vi "Sistema_Aquisicao.vi"() -> ()   [LabVIEW 2012]
uses:
  Global_Telescopio.vi
panel:
  out "error out":errorcluster
  out "ultimo valor 2":dbl format="%#_9g"
  out "ultimo valor":dbl format="%#_9g"
  out "ultimo comando":dbl
  in  "Case Constant\n(See Context Help)":bool=TRUE
  out "O Recebido":bool
  out "TimeoutAq":u32
  out "concatenated string":string
  out "Maq Satus":i32
  out "TX":string
  out "Serial Settings:Number of Bytes at Serial Port":u32
  out "Data rx Aquisição":string
  # "2"
  # "R -->Registra Centragem\nS -->Status\nO -->OffSet\nF ---> Foco"
  # "3"
  # "4"
  # "5"
  # "!"
  # "!"
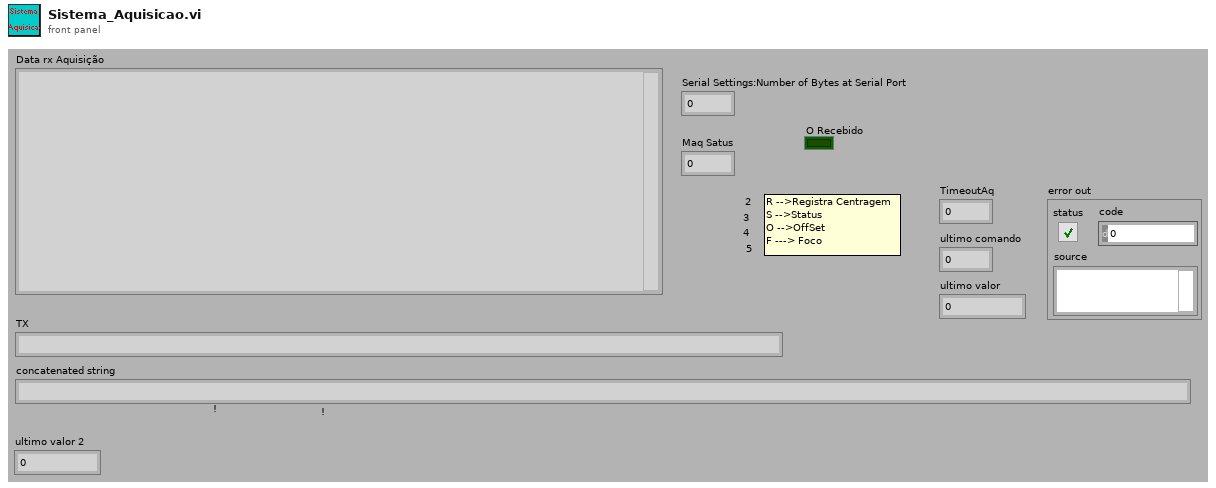
[diagram p1: front panel]
types:
  T1 = enum16{"open", "open or create", "create or replace", "create"}
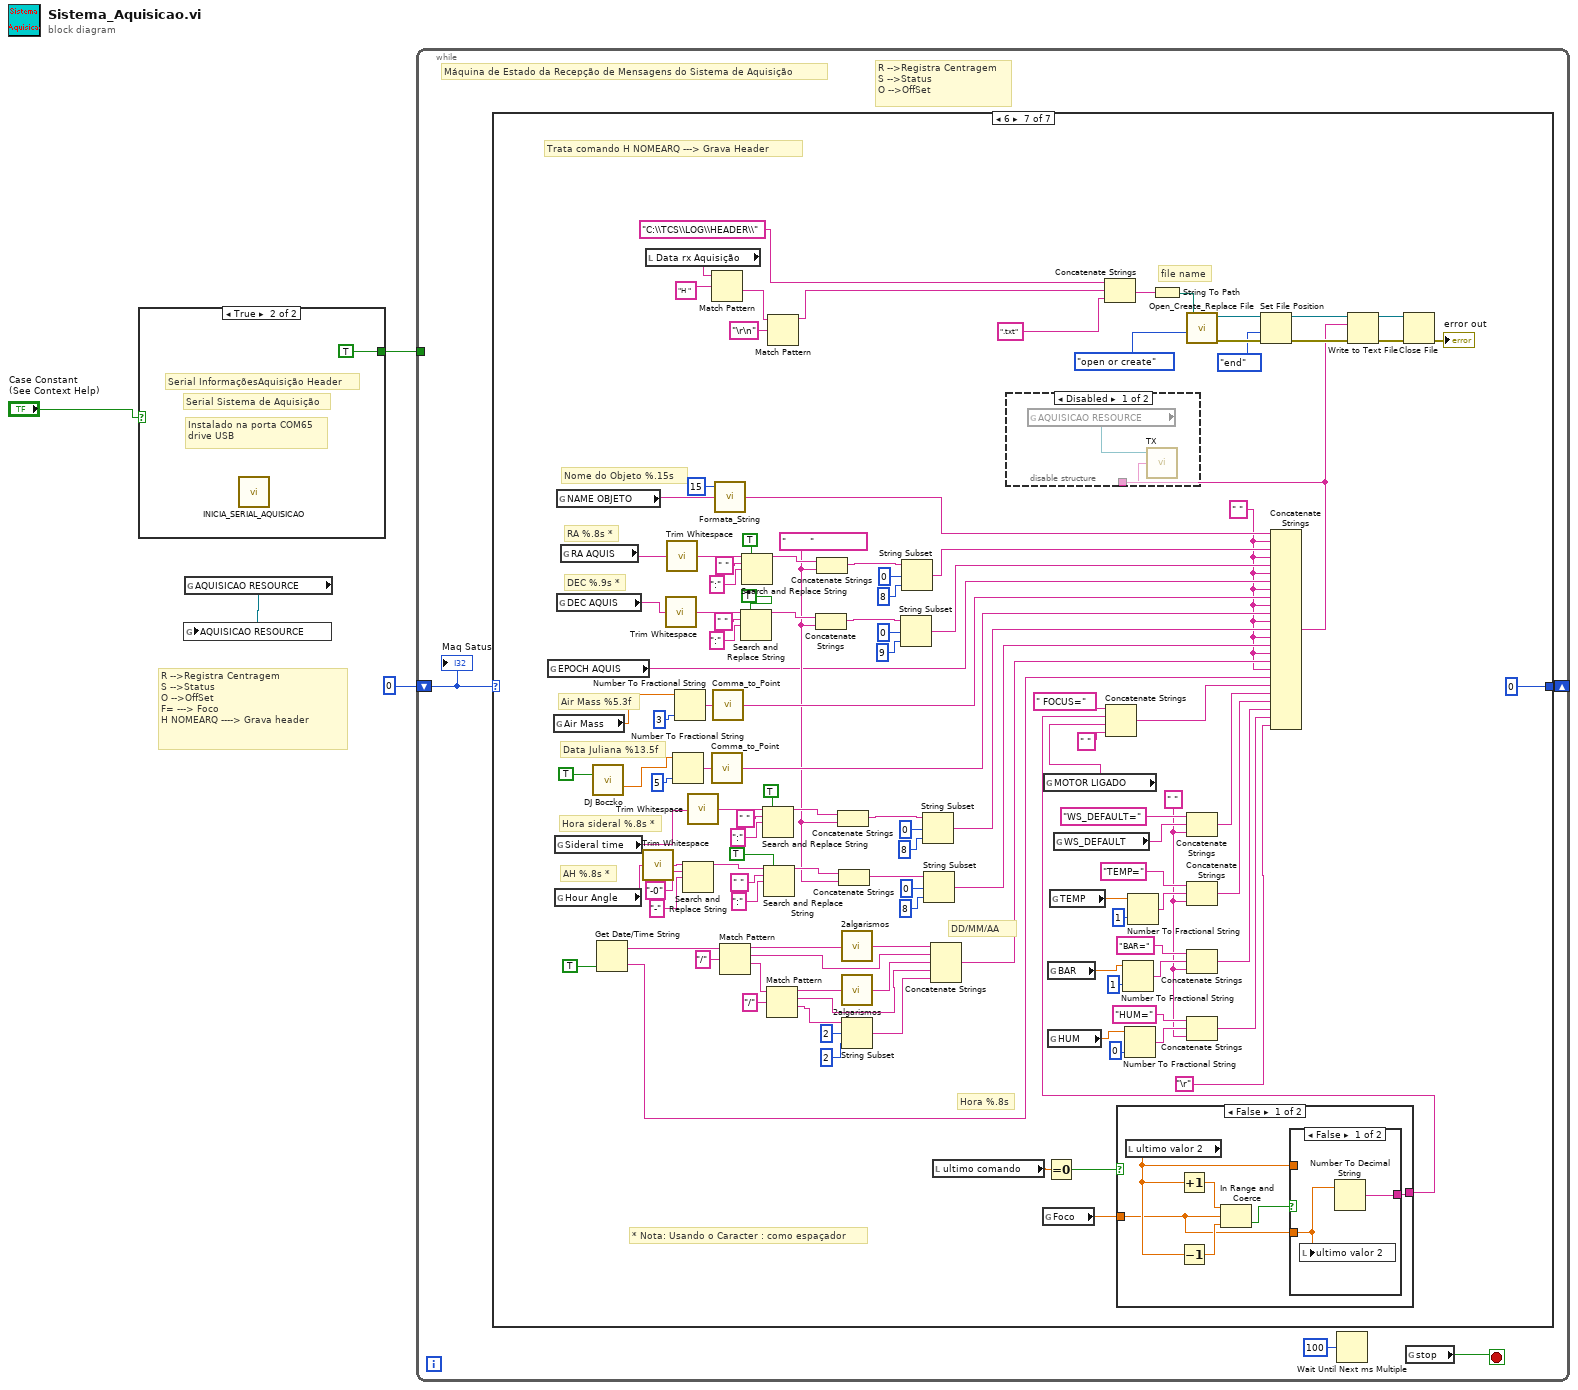
[diagram p0: block diagram]
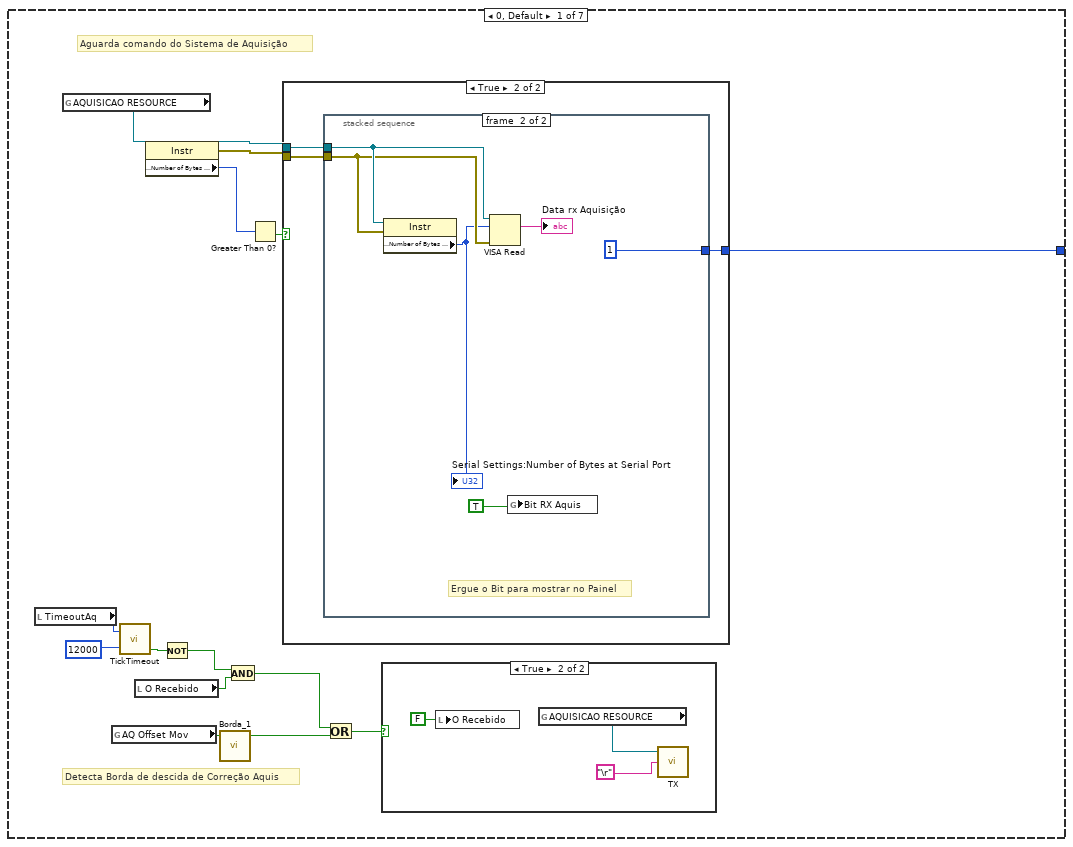
[diagram p3: hidden frame]
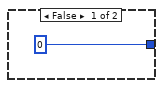
[diagram p5: hidden frame]
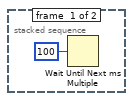
[diagram p6: hidden frame]
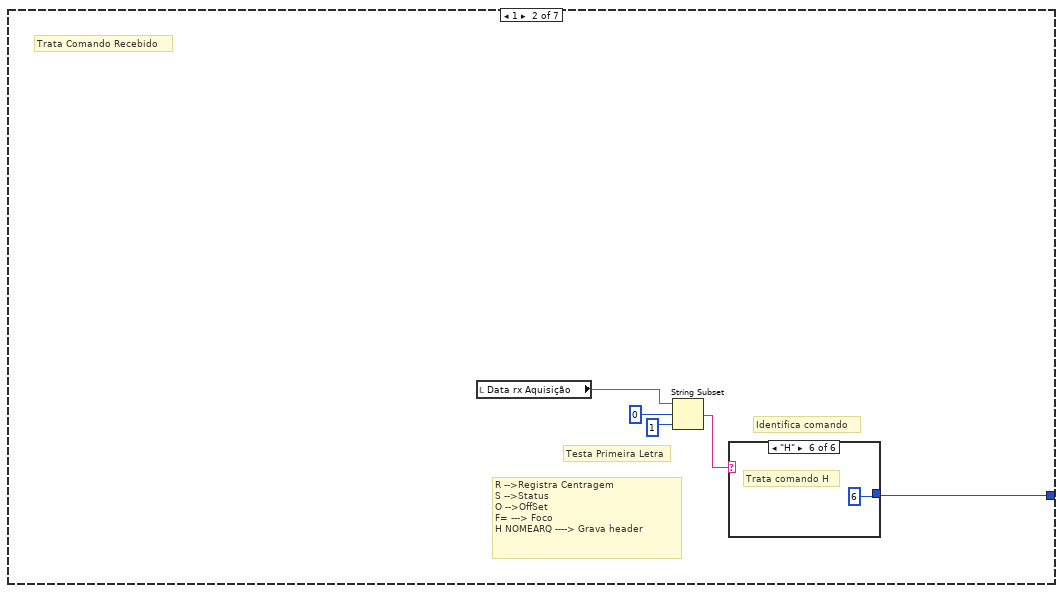
[diagram p7: hidden frame]
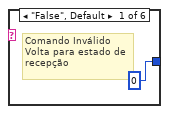
[diagram p8: hidden frame]
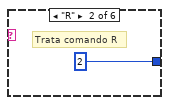
[diagram p9: hidden frame]
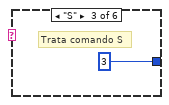
[diagram p10: hidden frame]
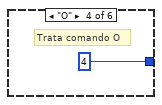
[diagram p11: hidden frame]
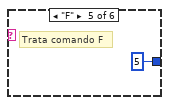
[diagram p12: hidden frame]
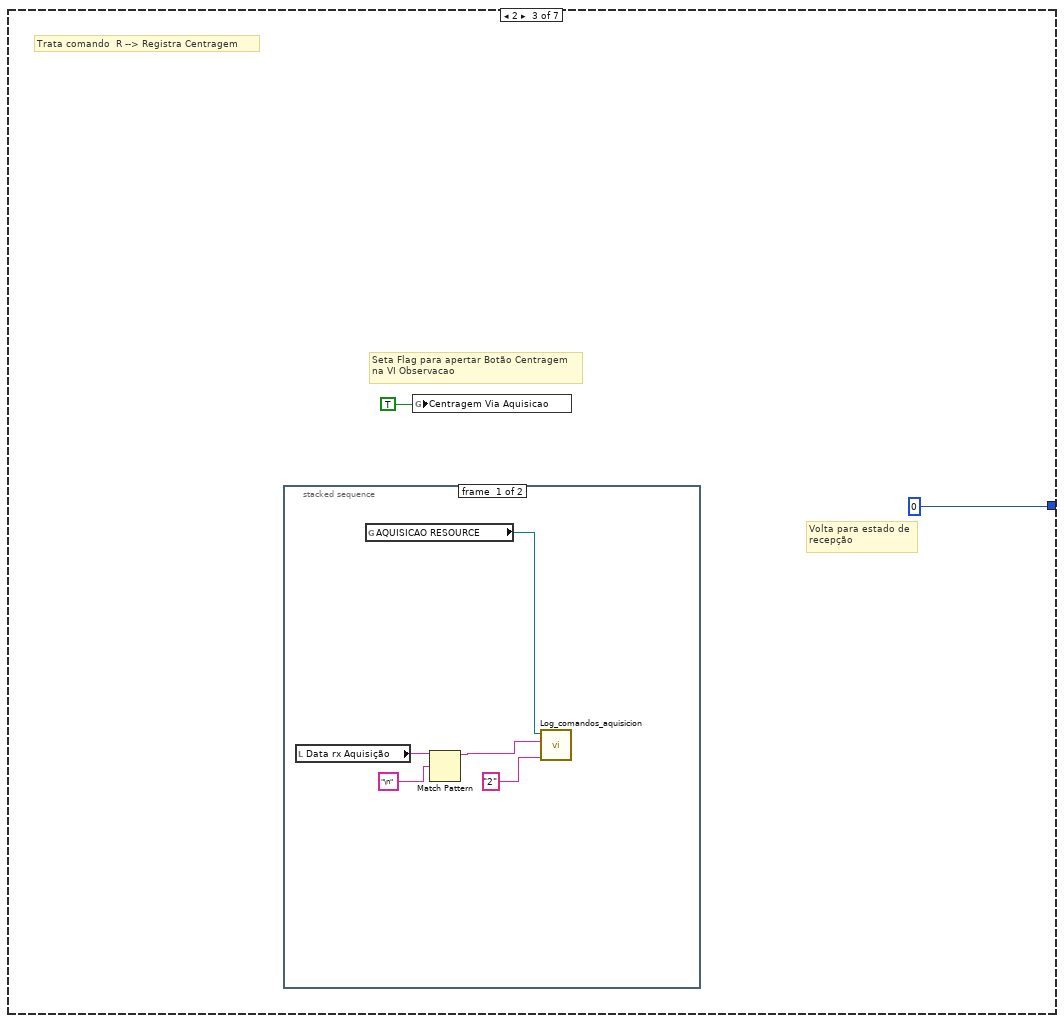
[diagram p13: hidden frame]
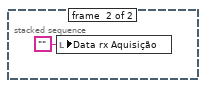
[diagram p14: hidden frame]
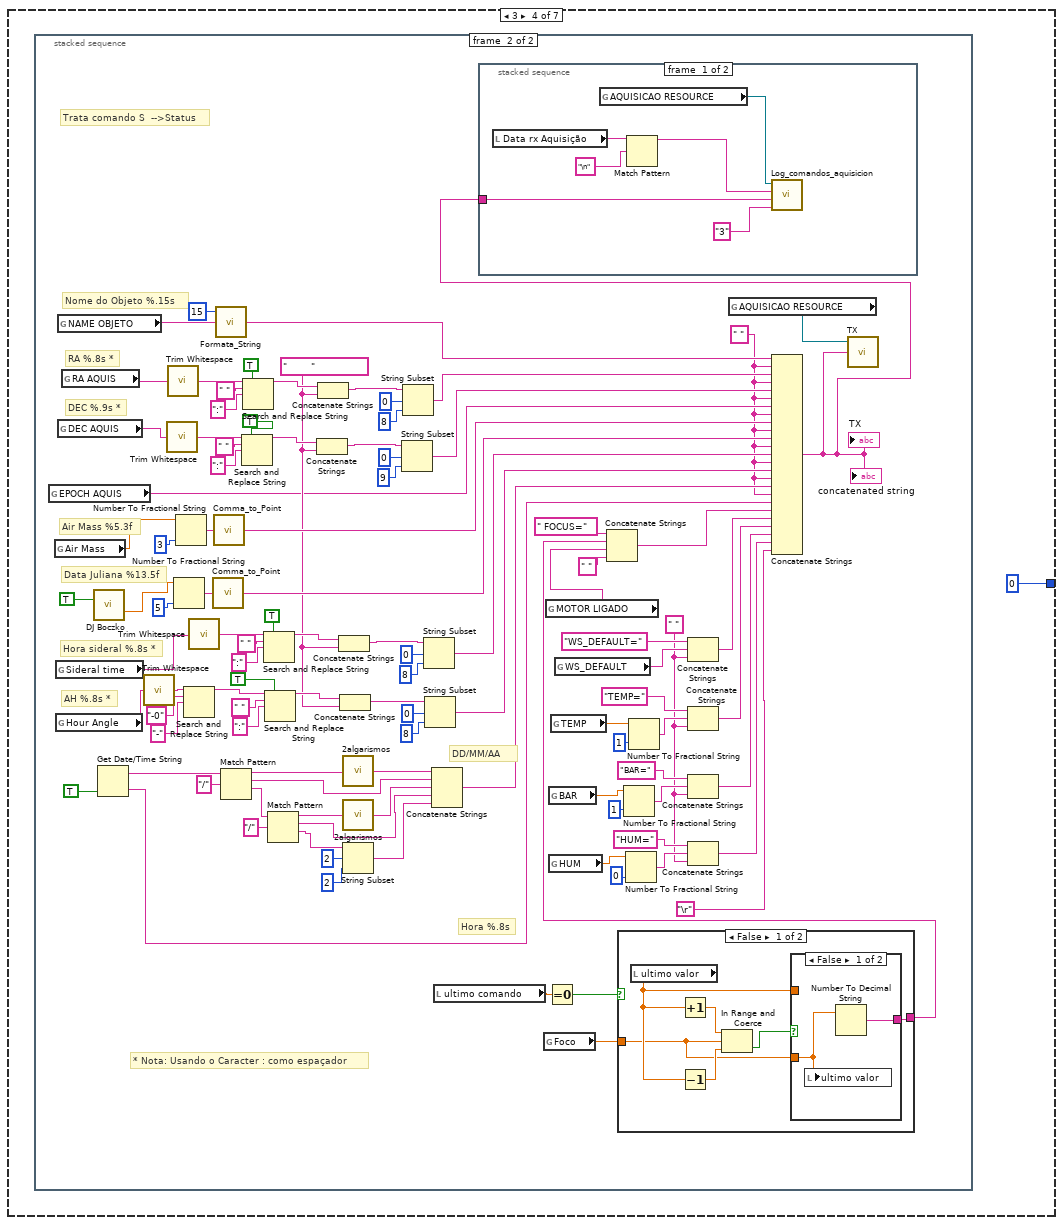
[diagram p15: hidden frame]
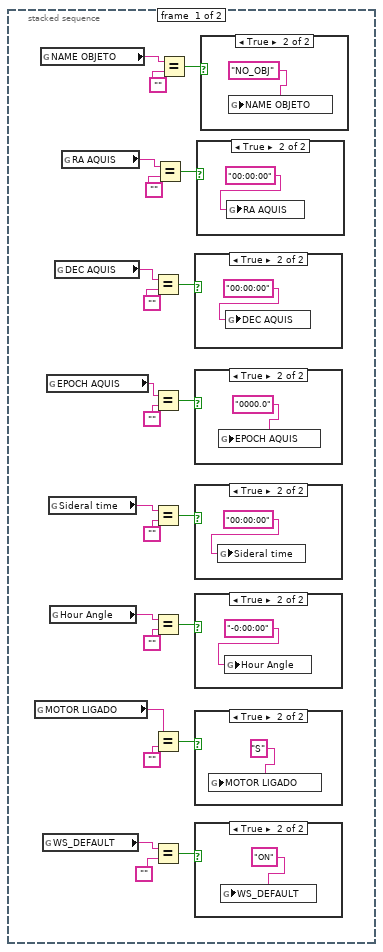
[diagram p16: hidden frame]
diagram:
  # "R -->Registra Centragem\nS -->Status\nO -->OffSet\nF= ---> Foco\nH NOMEARQ ----> Grava header"
  n1 = case shown="True" "Case Constant\n(See Context Help)" {
    tunnel: [_ TRUE] -> w2
    frame False {
    }
    frame True {
      # "Instalado na porta COM65\ndrive USB"
      # "Serial Sistema de Aquisição"
      # "Serial InformaçõesAquisição Header"
      n2 = call "INICIA_SERIAL_AQUISICAO.vi"() -> ()  [unwired: 1 in]
    }
  }
  n3 = global read "Global_Telescopio.vi" "AQUISICAO RESOURCE"() -> (w1:refnum<visa-resource-name>)
  n4 = global write "Global_Telescopio.vi" "AQUISICAO RESOURCE"(w1) -> ()
  n5 = while {
    shift-right: [w6] -> _
    shift-left: 0 -> [w7]
    tunnel: w2 -> [_]
    stop <- w9 stop-if-true
    # "R -->Registra Centragem\nS -->Status\nO -->OffSet"
    # "Máquina de Estado da Recepção de Mensagens do Sistema de Aquisição"
    n6 = case shown="6" w7 {
      tunnel: [w20 w39 0 0 0 0 0] -> w6
      frame 0, Default {
        # "Detecta Borda de descida de Correção Aquis"
        # "Aguarda comando do Sistema de Aquisição"
        n7 = local read "TimeoutAq"() -> (w12:u32)
        n8 = global read "Global_Telescopio.vi" "AQUISICAO RESOURCE"() -> (w19:refnum<visa-resource-name>)
        n9 = global read "Global_Telescopio.vi" "AQ Offset Mov"() -> (w17:bool)
        n10 = call "TickTimeout.vi"("msInicial"=w12, "msTimeout"=u32 12000) -> ("Timeout"=w13:bool)  [unwired: 2 out]
        n11 = local read "O Recebido"() -> (w15:bool)
        n12 = property class="Instr"(reference=w19) -> (reference out=w24:refnum<visa-resource-name>, error out=w23:errorcluster, "Serial Settings:Number of Bytes at Serial Port"=w22:u32)  [unwired: 1 in]
        n13 = Not(x=w13) -> (.not. x?=w11:bool)
        n14 = call "Borda_1.vi"("Entrada"=w17) -> ("Boolean"=w18:bool)  [unwired: 4 in]
        n15 = And(x=w11, y=w15) -> (x .and. y?=w10:bool)
        n16 = Greater Than 0?(x=w22) -> (x > 0?=w21:bool)
        n17 = case shown="True" w21 {
          tunnel: w24 -> [_ w31]
          tunnel: w23 -> [_ w30]
          tunnel: [0 w29] -> w20
          frame False {
          }
          frame True {
            n18 = stacked-sequence {
              tunnel: w31 -> [_ w38]
              tunnel: w30 -> [_ w37]
              tunnel: [_ 1] -> w29
              frame #0 {
                n19 = Wait Until Next ms Multiple(millisecond multiple=u32 100) -> ()  [unwired: 1 out]
              }
              frame #1 {
                # "Ergue o Bit para mostrar no Painel"
                n20 = property class="Instr"(reference=w38, error in=w37) -> ("Serial Settings:Number of Bytes at Serial Port"=w36:u32)  [unwired: 2 out]
                "Serial Settings:Number of Bytes at Serial Port" <- w36
                n21 = VISA Read(VISA resource name=w38, byte count=w36, error in (no error)=w37) -> (read buffer=→"Data rx Aquisição":string)  [unwired: 3 out]
                n22 = global write "Global_Telescopio.vi" "Bit RX Aquis"(TRUE) -> ()
              }
            }
          }
        }
        n23 = Or(x=w10, y=w18) -> (x .or. y?=w16:bool)
        n24 = case shown="True" w16 {
          frame False {
          }
          frame True {
            n25 = local write "O Recebido"(FALSE ("O Recebido")) -> ()
            n26 = global read "Global_Telescopio.vi" "AQUISICAO RESOURCE"() -> (w27:refnum<visa-resource-name>)
            n27 = call "TX.vi"("tx_buf"="\r", "VISA resource name"=w27) -> ()  [unwired: 1 in, 3 out]
          }
        }
      }
      frame 1 {
        # "R -->Registra Centragem\nS -->Status\nO -->OffSet\nF= ---> Foco\nH NOMEARQ ----> Grava header"
        # "Testa Primeira Letra"
        # "Identifica comando"
        # "Trata Comando Recebido"
        n28 = local read "Data rx Aquisição"() -> (w40:string)
        n29 = String Subset(string=w40, offset (0)=0, length (rest)=1 ("length (rest)")) -> (substring=w43:string)
        n30 = case shown="\"H\"" w43 {
          tunnel: [0 2 3 4 5 6] -> w39
          frame "False", Default {
            # "Comando Inválido\nVolta para estado de\nrecepção"
          }
          frame "R" {
            # "Trata comando R"
          }
          frame "S" {
            # "Trata comando S"
          }
          frame "O" {
            # "Trata comando O"
          }
          frame "F" {
            # "Trata comando F"
          }
          frame "H" {
            # "Trata comando H"
          }
        }
      }
      frame 2 {
        # "Seta Flag para apertar Botão Centragem\nna VI Observacao"
        # "Trata comando  R --> Registra Centragem"
        # "Volta para estado de\nrecepção"
        n31 = stacked-sequence {
          frame #0 {
            n32 = local read "Data rx Aquisição"() -> (w53:string)
            n33 = global read "Global_Telescopio.vi" "AQUISICAO RESOURCE"() -> (w56:refnum<visa-resource-name>)
            n34 = Match Pattern(string=w53, regular expression="\n") -> (before substring=w52:string)  [unwired: 1 in, 3 out]
            n35 = call "Log_comandos_aquisicion.vi"("Estado"="2", "string de comando"=w52, "Porta"=w56) -> ()  [unwired: 9 in]
          }
          frame #1 {
            n36 = local write "Data rx Aquisição"("") -> ()
          }
        }
        n37 = global write "Global_Telescopio.vi" "Centragem Via Aquisicao"(TRUE ("Comunicaçao ok guider")) -> ()
      }
      frame 3 {
        n38 = stacked-sequence {
          frame #0 {
            n39 = global read "Global_Telescopio.vi" "MOTOR LIGADO"() -> (w79:string)
            n40 = global read "Global_Telescopio.vi" "NAME OBJETO"() -> (w60:string)
            n41 = global read "Global_Telescopio.vi" "WS_DEFAULT"() -> (w81:string)
            n42 = global read "Global_Telescopio.vi" "EPOCH AQUIS"() -> (w69:string)
            n43 = global read "Global_Telescopio.vi" "Sideral time"() -> (w71:string)
            n44 = global read "Global_Telescopio.vi" "Hour Angle"() -> (w76:string)
            n45 = global read "Global_Telescopio.vi" "DEC AQUIS"() -> (w67:string)
            n46 = global read "Global_Telescopio.vi" "RA AQUIS"() -> (w64:string)
            n47 = Equal?(x=w67, y="") -> (x = y?=w66:bool)
            n48 = Equal?(x=w69, y="") -> (x = y?=w68:bool)
            n49 = Equal?(x=w71, y="") -> (x = y?=w70:bool)
            n50 = Equal?(x=w76, y="") -> (x = y?=w72:bool)
            n51 = Equal?(x=w79, y="") -> (x = y?=w78:bool)
            n52 = Equal?(x=w81, y="") -> (x = y?=w80:bool)
            n53 = Equal?(x=w64, y="") -> (x = y?=w62:bool)
            n54 = Equal?(x=w60, y="") -> (x = y?=w61:bool)
            n55 = case shown="True" w66 {
              frame False {
              }
              frame True {
                n56 = global write "Global_Telescopio.vi" "DEC AQUIS"("00:00:00" ("NAME OBJETO")) -> ()
              }
            }
            n57 = case shown="True" w68 {
              frame False {
              }
              frame True {
                n58 = global write "Global_Telescopio.vi" "EPOCH AQUIS"("0000.0" ("NAME OBJETO")) -> ()
              }
            }
            n59 = case shown="True" w70 {
              frame False {
              }
              frame True {
                n60 = global write "Global_Telescopio.vi" "Sideral time"("00:00:00" ("NAME OBJETO")) -> ()
              }
            }
            n61 = case shown="True" w72 {
              frame False {
              }
              frame True {
                n62 = global write "Global_Telescopio.vi" "Hour Angle"("-0:00:00" ("NAME OBJETO")) -> ()
              }
            }
            n63 = case shown="True" w78 {
              frame False {
              }
              frame True {
                n64 = global write "Global_Telescopio.vi" "MOTOR LIGADO"("S") -> ()
              }
            }
            n65 = case shown="True" w80 {
              frame False {
              }
              frame True {
                n66 = global write "Global_Telescopio.vi" "WS_DEFAULT"("ON" ("Hora a ser Procurada")) -> ()
              }
            }
            n67 = case shown="True" w62 {
              frame False {
              }
              frame True {
                n68 = global write "Global_Telescopio.vi" "RA AQUIS"("00:00:00" ("NAME OBJETO")) -> ()
              }
            }
            n69 = case shown="True" w61 {
              frame False {
              }
              frame True {
                n70 = global write "Global_Telescopio.vi" "NAME OBJETO"("NO_OBJ" ("NAME OBJETO")) -> ()
              }
            }
          }
          frame #1 {
            w96 = " " ("string")
            w151 = "        " ("string")
            w105 = " "
            # "* Nota: Usando o Caracter : como espaçador"
            # "Hora %.8s"
            # "DD/MM/AA"
            # "AH %.8s *"
            # "Hora sideral %.8s *"
            # "Data Juliana %13.5f"
            # "Air Mass %5.3f"
            # "DEC %.9s *"
            # "RA %.8s *"
            # "Nome do Objeto %.15s"
            # "Trata comando S  -->Status"
            n71 = global read "Global_Telescopio.vi" "EPOCH AQUIS"() -> (w121:string)
            n72 = global read "Global_Telescopio.vi" "Air Mass"() -> (w130:dbl)
            n73 = global read "Global_Telescopio.vi" "Sideral time"() -> (w160:string)
            n74 = global read "Global_Telescopio.vi" "Hour Angle"() -> (w122:string)
            n75 = global read "Global_Telescopio.vi" "NAME OBJETO"() -> (w129:string)
            n76 = global read "Global_Telescopio.vi" "DEC AQUIS"() -> (w177:string)
            n77 = global read "Global_Telescopio.vi" "RA AQUIS"() -> (w192:string)
            n78 = call "DJ Boczko.vi"("TRUE = Hora Local\nFALSE = UT"=TRUE ("TRUE = Hora Local\nFALSE = UT")) -> ("Dia Juliano"=w170:dbl)  [unwired: 6 in, 8 out]
            n79 = Get Date/Time String(want seconds? (F)=TRUE) -> (date string=w148:string, time string=w133:string)  [unwired: 2 in]
            n80 = call <vilib>:"Trim Whitespace.vi"("string"=w122) -> ("trimmed string"=w123:string)  [unwired: 1 in]
            n81 = call <vilib>:"Trim Whitespace.vi"("string"=w177) -> ("trimmed string"=w180:string)  [unwired: 1 in]
            n82 = call <vilib>:"Trim Whitespace.vi"("string"=w192) -> ("trimmed string"=w191:string)  [unwired: 1 in]
            n83 = Number To Fractional String(number=w170, precision (6)=i16 5) -> (F-format string=w169:string)  [unwired: 2 in]
            n84 = Number To Fractional String(number=w130, precision (6)=i16 3) -> (F-format string=w173:string)  [unwired: 2 in]
            n85 = Search and Replace String(input string=w123, search string="-0", replace string="-" ("replace string (\"\")")) -> (result string=w124:string)  [unwired: 5 in, 3 out]
            n86 = call <vilib>:"Trim Whitespace.vi"("string"=w160) -> ("trimmed string"=w163:string)  [unwired: 1 in]
            n87 = call "Comma_to_Point.vi"("Lat_A"=w169) -> ("Saída"=w168:string)
            n88 = call "Comma_to_Point.vi"("Lat_A"=w173) -> ("Saída"=w172:string)
            n89 = call "Formata_String.vi"("entrada"=w129, "Num de Caracteres"=15) -> ("saida"=w127:string)  [unwired: 3 in]
            n90 = Match Pattern(string=w148, regular expression="/") -> (before substring=w144:string, match substring=w138:string, after substring=w145:string)  [unwired: 1 in, 1 out]
            n91 = Search and Replace String(replace all?=TRUE ("replace all? (F)"), input string=w180, search string=" ", replace string=":" ("replace string (\"\")")) -> (result string=w183:string)  [unwired: 4 in, 3 out]
            n92 = Search and Replace String(replace all?=TRUE ("replace all? (F)"), input string=w191, search string=" ", replace string=":" ("replace string (\"\")")) -> (result string=w187:string)  [unwired: 4 in, 3 out]
            n93 = Search and Replace String(replace all?=TRUE ("replace all? (F)"), input string=w163, search string=" ", replace string=":" ("replace string (\"\")")) -> (result string=w166:string)  [unwired: 4 in, 3 out]
            n94 = Search and Replace String(replace all?=TRUE ("replace all? (F)"), input string=w124, search string=" ", replace string=":" ("replace string (\"\")")) -> (result string=w153:string)  [unwired: 4 in, 3 out]
            n95 = Match Pattern(string=w145, regular expression="/") -> (before substring=w143:string, match substring=w136:string, after substring=w142:string)  [unwired: 1 in, 1 out]
            n96 = Concatenate Strings(w183, w151) -> (w184:string)
            n97 = Concatenate Strings(w187, w151) -> (w186:string)
            n98 = Concatenate Strings(w166, w151) -> (w167:string)
            n99 = Concatenate Strings(w153, w151) -> (w152:string)
            n100 = call "2algarismos.vi"("entrada"=w144) -> ("saida"=w139:string)
            n101 = call "2algarismos.vi"("entrada"=w143) -> ("saida"=w137:string)
            n102 = String Subset(string=w142, offset (0)=2, length (rest)=2 ("length (rest)")) -> (substring=w135:string)
            n103 = String Subset(string=w184, offset (0)=0, length (rest)=9 ("length (rest)")) -> (substring=w176:string)
            n104 = String Subset(string=w186, offset (0)=0, length (rest)=8 ("length (rest)")) -> (substring=w185:string)
            n105 = String Subset(string=w167, offset (0)=0, length (rest)=8 ("length (rest)")) -> (substring=w158:string)
            n106 = String Subset(string=w152, offset (0)=0, length (rest)=8 ("length (rest)")) -> (substring=w150:string)
            n107 = Concatenate Strings(w139, w138, w137, w136, w135) -> (w134:string)
            n108 = local read "ultimo comando"() -> (w120:dbl)
            n109 = global read "Global_Telescopio.vi" "Foco"() -> (w114:dbl)
            n110 = global read "Global_Telescopio.vi" "MOTOR LIGADO"() -> (w113:string)
            n111 = Equal To 0?(x=w120) -> (x = 0?=w119:bool)
            n112 = global read "Global_Telescopio.vi" "BAR"() -> (w107:dbl)
            n113 = global read "Global_Telescopio.vi" "HUM"() -> (w106:dbl)
            n114 = global read "Global_Telescopio.vi" "TEMP"() -> (w111:dbl)
            n115 = global read "Global_Telescopio.vi" "WS_DEFAULT"() -> (w103:string)
            n116 = case shown="False" w119 {
              tunnel: [w204 w214] -> w117
              tunnel: w114 -> [w203 w213]
              frame False {
                n117 = local read "ultimo valor"() -> (w205:dbl)
                n118 = Increment(x=w205) -> (x+1=w207:dbl)
                n119 = Decrement(x=w205) -> (x-1=w206:dbl)
                n120 = In Range and Coerce(upper limit=w207, x=w203, lower limit=w206) -> (In Range?=w208:bool)  [unwired: 1 out]
                n121 = case shown="False" w208 {
                  tunnel: w205 -> [_ w212]
                  tunnel: [w210 w211] -> w204
                  tunnel: w203 -> [w209 _]
                  frame False {
                    n122 = local write "ultimo valor"(w209) -> ()
                    n123 = Number To Decimal String(number=w209) -> (decimal integer string=w210:string)  [unwired: 1 in]
                  }
                  frame True {
                    n124 = Number To Decimal String(number=w212) -> (decimal integer string=w211:string)  [unwired: 1 in]
                  }
                }
              }
              frame True {
                n125 = Number To Decimal String(number=w213) -> (decimal integer string=w214:string)  [unwired: 1 in]
                "ultimo valor" <- w213
              }
            }
            n126 = Concatenate Strings(" FOCUS=" ("string"), w117, w113, " " ("string")) -> (w115:string)
            n127 = Number To Fractional String(number=w107, precision (6)=i16 1) -> (F-format string=w98:string)  [unwired: 2 in]
            n128 = Number To Fractional String(number=w106, precision (6)=i16 0) -> (F-format string=w97:string)  [unwired: 2 in]
            n129 = Number To Fractional String(number=w111, precision (6)=i16 1) -> (F-format string=w100:string)  [unwired: 2 in]
            n130 = Concatenate Strings("WS_DEFAULT=" ("string"), w103, w96) -> (w95:string)
            n131 = Concatenate Strings("TEMP=" ("string"), w100, w96) -> (w94:string)
            n132 = Concatenate Strings("BAR=" ("string"), w98, w96) -> (w93:string)
            n133 = Concatenate Strings("HUM=" ("string"), w97, w96) -> (w92:string)
            n134 = global read "Global_Telescopio.vi" "AQUISICAO RESOURCE"() -> (w195:refnum<visa-resource-name>)
            n135 = Concatenate Strings(w127, w105, w185, w105, w176, w105, w121, w105, w172, w105, w168, w105, w158, w105, w150, w105, w134, w105, w133, w115, w95, w94, w93, w92, "\r") -> (w118:string)
            "TX" <- w118
            "concatenated string" <- w118
            n136 = stacked-sequence {
              tunnel: w118 -> [w199 _]
              frame #0 {
                n137 = local read "Data rx Aquisição"() -> (w198:string)
                n138 = global read "Global_Telescopio.vi" "AQUISICAO RESOURCE"() -> (w201:refnum<visa-resource-name>)
                n139 = Match Pattern(string=w198, regular expression="\n") -> (before substring=w196:string)  [unwired: 1 in, 3 out]
                n140 = call "Log_comandos_aquisicion.vi"("Estado"="3", "string de Resposta"=w199, "string de comando"=w196, "Porta"=w201) -> ()  [unwired: 8 in]
              }
              frame #1 {
                n141 = local write "Data rx Aquisição"("") -> ()
              }
            }
            n142 = call "TX.vi"("tx_buf"=w118, "VISA resource name"=w195) -> ()  [unwired: 1 in, 3 out]
          }
        }
      }
      frame 4 {
        # "Trata comando O  -->OffSet"
        n143 = local read "Data rx Aquisição"() -> (w217:string)
        n144 = String Subset(string=w217, offset (0)=2, length (rest)=1 ("length (rest)")) -> (substring=w226:string)
        n145 = String Subset(string=w217, offset (0)=3, length (rest)=4 ("length (rest)")) -> (substring=w233:string)
        n146 = String Subset(string=w217, offset (0)=8, length (rest)=1 ("length (rest)")) -> (substring=w225:string)
        n147 = String Subset(string=w217, offset (0)=1, length (rest)=1 ("length (rest)")) -> (substring=w219:string)
        n148 = String Subset(string=w217, offset (0)=9, length (rest)=4 ("length (rest)")) -> (substring=w232:string)
        n149 = Fract/Exp String To Number(use system decimal point (T)=FALSE, string=w233) -> (number=w222:dbl)  [unwired: 2 in, 1 out]
        n150 = Fract/Exp String To Number(use system decimal point (T)=FALSE, string=w232) -> (number=w220:dbl)  [unwired: 2 in, 1 out]
        n151 = case shown="\"N\"" w226 {
          tunnel: [0.0 ("PreciseOffsetDEC 2") 1.0 ("PreciseOffsetDEC 2") -1.0 ("PreciseOffsetDEC 2")] -> w223
          frame " ", Default {
          }
          frame "N" {
          }
          frame "S" {
          }
        }
        n152 = case shown="\"E\"" w225 {
          tunnel: [0.0 ("PreciseOffsetDEC 2") 1.0 ("PreciseOffsetDEC 2") -1.0 ("PreciseOffsetDEC 2")] -> w221
          frame " ", Default {
          }
          frame "W" {
          }
          frame "E" {
          }
        }
        n153 = call "Salva_comando_Apend.vi"("String"=w217, "file name p/ exell"="C:\\TCS\\LOG\\Comando_O_Aquisicao.txt") -> ()  [unwired: 4 in]
        n154 = Multiply(x=w223, y=w221) -> (x*y=w227:dbl)
        n155 = Equal To 0?(x=w227) -> (x = 0?=w224:bool)
        n156 = case shown="False" w224 {
          tunnel: w223 -> [w260 _]
          tunnel: w222 -> [w259 _]
          tunnel: w221 -> [w258 _]
          tunnel: w220 -> [w257 _]
          tunnel: w219 -> [w255 _]
          tunnel: [TRUE ("Correção Aquis") FALSE ("Correção Aquis")] -> w218
          tunnel: ["" ""] -> w215
          frame False {
            n157 = Multiply(x=w260, y=w259) -> (x*y=w252:dbl)
            n158 = Multiply(x=w258, y=w257) -> (x*y=w256:dbl)
            n159 = case shown="\"1\"" w255 {
              tunnel: [1.0 ("PreciseOffsetDEC 2") w262] -> w254
              frame "0", Default {
              }
              frame "1" {
                n160 = global read "Global_Telescopio.vi" "delta_now"() -> (w263:dbl)
                n161 = Cosine(x=w263) -> (cos(x)=w264:dbl)
                n162 = Absolute Value(x=w264) -> (abs(x)=w262:dbl)
              }
            }
            n163 = Divide(x=w256, y=w254) -> (x/y=w253:dbl)
            n164 = global write "Global_Telescopio.vi" "aquis_asc"(w253) -> ()
            n165 = global write "Global_Telescopio.vi" "aquis_dec"(w252) -> ()
            n166 = call "TickTimeout.vi"() -> ("msTick"=→"TimeoutAq":u32)  [unwired: 2 in, 2 out]
          }
          frame True {
          }
        }
        "O Recebido" <- w218
        n167 = stacked-sequence {
          tunnel: w215 -> [_ w248]
          frame #0 {
            n168 = local read "Data rx Aquisição"() -> (w244:string)
            n169 = global read "Global_Telescopio.vi" "AQUISICAO RESOURCE"() -> (w247:refnum<visa-resource-name>)
            n170 = Match Pattern(string=w244, regular expression="\n") -> (before substring=w243:string)  [unwired: 1 in, 3 out]
            n171 = call "Log_comandos_aquisicion.vi"("Estado"="4", "string de comando"=w243, "Porta"=w247) -> ()  [unwired: 9 in]
          }
          frame #1 {
            n172 = local write "Data rx Aquisição"(w248) -> ()
          }
        }
        n173 = global write "Global_Telescopio.vi" "Correção Aquis"(w218) -> ()
      }
      frame 5 {
        # "Trata comando F ---> Trata o comando de foco vindo do computador de aquisição"
        n174 = local read "Data rx Aquisição"() -> (w281:string)
        n175 = Match Pattern(string=w281, regular expression="=") -> (after substring=w279:string)  [unwired: 1 in, 3 out]
        n176 = Fract/Exp String To Number(string=w279) -> (number=w275:dbl)  [unwired: 3 in, 1 out]
        n177 = In Range and Coerce(upper limit=2012.0, x=w275, lower limit=1.0) -> (In Range?=w276:bool)  [unwired: 1 out]
        n178 = case shown="True" w276 {
          tunnel: w275 -> [_ w291]
          tunnel: ["" ""] -> w273
          frame False {
          }
          frame True {
            n179 = case shown="True" TRUE {
              tunnel: ["stop" ("Comando") "go" ("Comando")] -> w290
              frame False {
              }
              frame True {
                n180 = call "TX focus FOCO.vi"("Comando"="def", "Setpoint"=20.0) -> ()  [unwired: 11 in, 3 out]
              }
            }
            n181 = call "TX focus FOCO.vi"("Comando"=w290, "Setpoint"=w291) -> ()  [unwired: 11 in, 3 out]
            "ultimo comando" <- w291
          }
        }
        n182 = stacked-sequence {
          tunnel: w273 -> [_ w287]
          frame #0 {
            n183 = local read "Data rx Aquisição"() -> (w283:string)
            n184 = global read "Global_Telescopio.vi" "AQUISICAO RESOURCE"() -> (w286:refnum<visa-resource-name>)
            n185 = Match Pattern(string=w283, regular expression="\n") -> (before substring=w282:string)  [unwired: 1 in, 3 out]
            n186 = call "Log_comandos_aquisicion.vi"("Estado"="5", "string de comando"=w282, "Porta"=w286) -> ()  [unwired: 9 in]
          }
          frame #1 {
            n187 = local write "Data rx Aquisição"(w287) -> ()
          }
        }
      }
      frame 6 {
        w321 = " " ("string")
        w375 = "        " ("string")
        w330 = " "
        # "file name"
        # "* Nota: Usando o Caracter : como espaçador"
        # "Hora %.8s"
        # "DD/MM/AA"
        # "AH %.8s *"
        # "Hora sideral %.8s *"
        # "Data Juliana %13.5f"
        # "Air Mass %5.3f"
        # "DEC %.9s *"
        # "RA %.8s *"
        # "Nome do Objeto %.15s"
        # "Trata comando H NOMEARQ ---> Grava Header"
        n188 = global read "Global_Telescopio.vi" "EPOCH AQUIS"() -> (w345:string)
        n189 = global read "Global_Telescopio.vi" "Air Mass"() -> (w354:dbl)
        n190 = global read "Global_Telescopio.vi" "Sideral time"() -> (w384:string)
        n191 = global read "Global_Telescopio.vi" "Hour Angle"() -> (w346:string)
        n192 = global read "Global_Telescopio.vi" "NAME OBJETO"() -> (w353:string)
        n193 = global read "Global_Telescopio.vi" "DEC AQUIS"() -> (w401:string)
        n194 = global read "Global_Telescopio.vi" "RA AQUIS"() -> (w416:string)
        n195 = call "DJ Boczko.vi"("TRUE = Hora Local\nFALSE = UT"=TRUE ("TRUE = Hora Local\nFALSE = UT")) -> ("Dia Juliano"=w394:dbl)  [unwired: 6 in, 8 out]
        n196 = Get Date/Time String(want seconds? (F)=TRUE) -> (date string=w372:string, time string=w357:string)  [unwired: 2 in]
        n197 = call <vilib>:"Trim Whitespace.vi"("string"=w346) -> ("trimmed string"=w347:string)  [unwired: 1 in]
        n198 = local read "Data rx Aquisição"() -> (w315:string)
        n199 = call <vilib>:"Trim Whitespace.vi"("string"=w401) -> ("trimmed string"=w404:string)  [unwired: 1 in]
        n200 = call <vilib>:"Trim Whitespace.vi"("string"=w416) -> ("trimmed string"=w415:string)  [unwired: 1 in]
        n201 = Number To Fractional String(number=w394, precision (6)=i16 5) -> (F-format string=w393:string)  [unwired: 2 in]
        n202 = Number To Fractional String(number=w354, precision (6)=i16 3) -> (F-format string=w397:string)  [unwired: 2 in]
        n203 = Search and Replace String(input string=w347, search string="-0", replace string="-" ("replace string (\"\")")) -> (result string=w348:string)  [unwired: 5 in, 3 out]
        n204 = call <vilib>:"Trim Whitespace.vi"("string"=w384) -> ("trimmed string"=w387:string)  [unwired: 1 in]
        n205 = Match Pattern(string=w315, regular expression="H ") -> (after substring=w300:string)  [unwired: 1 in, 3 out]
        n206 = call "Comma_to_Point.vi"("Lat_A"=w393) -> ("Saída"=w392:string)
        n207 = call "Comma_to_Point.vi"("Lat_A"=w397) -> ("Saída"=w396:string)
        n208 = call "Formata_String.vi"("entrada"=w353, "Num de Caracteres"=15) -> ("saida"=w351:string)  [unwired: 3 in]
        n209 = Match Pattern(string=w372, regular expression="/") -> (before substring=w368:string, match substring=w362:string, after substring=w369:string)  [unwired: 1 in, 1 out]
        n210 = Search and Replace String(replace all?=TRUE ("replace all? (F)"), input string=w404, search string=" ", replace string=":" ("replace string (\"\")")) -> (result string=w407:string)  [unwired: 4 in, 3 out]
        n211 = Search and Replace String(replace all?=TRUE ("replace all? (F)"), input string=w415, search string=" ", replace string=":" ("replace string (\"\")")) -> (result string=w411:string)  [unwired: 4 in, 3 out]
        n212 = Search and Replace String(replace all?=TRUE ("replace all? (F)"), input string=w387, search string=" ", replace string=":" ("replace string (\"\")")) -> (result string=w390:string)  [unwired: 4 in, 3 out]
        n213 = Search and Replace String(replace all?=TRUE ("replace all? (F)"), input string=w348, search string=" ", replace string=":" ("replace string (\"\")")) -> (result string=w377:string)  [unwired: 4 in, 3 out]
        n214 = Match Pattern(string=w369, regular expression="/") -> (before substring=w367:string, match substring=w360:string, after substring=w366:string)  [unwired: 1 in, 1 out]
        n215 = Match Pattern(string=w300, regular expression="\r\n") -> (before substring=w298:string)  [unwired: 1 in, 3 out]
        n216 = Concatenate Strings(w407, w375) -> (w408:string)
        n217 = Concatenate Strings(w411, w375) -> (w410:string)
        n218 = Concatenate Strings(w390, w375) -> (w391:string)
        n219 = Concatenate Strings(w377, w375) -> (w376:string)
        n220 = call "2algarismos.vi"("entrada"=w368) -> ("saida"=w363:string)
        n221 = call "2algarismos.vi"("entrada"=w367) -> ("saida"=w361:string)
        n222 = String Subset(string=w366, offset (0)=2, length (rest)=2 ("length (rest)")) -> (substring=w359:string)
        n223 = String Subset(string=w408, offset (0)=0, length (rest)=9 ("length (rest)")) -> (substring=w400:string)
        n224 = String Subset(string=w410, offset (0)=0, length (rest)=8 ("length (rest)")) -> (substring=w409:string)
        n225 = String Subset(string=w391, offset (0)=0, length (rest)=8 ("length (rest)")) -> (substring=w382:string)
        n226 = String Subset(string=w376, offset (0)=0, length (rest)=8 ("length (rest)")) -> (substring=w374:string)
        n227 = Concatenate Strings(w363, w362, w361, w360, w359) -> (w358:string)
        n228 = local read "ultimo comando"() -> (w344:dbl)
        n229 = global read "Global_Telescopio.vi" "Foco"() -> (w339:dbl)
        n230 = global read "Global_Telescopio.vi" "MOTOR LIGADO"() -> (w338:string)
        n231 = Equal To 0?(x=w344) -> (x = 0?=w343:bool)
        n232 = global read "Global_Telescopio.vi" "BAR"() -> (w332:dbl)
        n233 = global read "Global_Telescopio.vi" "HUM"() -> (w331:dbl)
        n234 = global read "Global_Telescopio.vi" "TEMP"() -> (w336:dbl)
        n235 = global read "Global_Telescopio.vi" "WS_DEFAULT"() -> (w328:string)
        n236 = Concatenate Strings("C:\\TCS\\LOG\\HEADER\\" ("string"), w298, ".txt" ("string")) -> (w305:string)
        n237 = case shown="False" w343 {
          tunnel: [w423 w433] -> w342
          tunnel: w339 -> [w422 w432]
          frame False {
            n238 = local read "ultimo valor 2"() -> (w424:dbl)
            n239 = Increment(x=w424) -> (x+1=w426:dbl)
            n240 = Decrement(x=w424) -> (x-1=w425:dbl)
            n241 = In Range and Coerce(upper limit=w426, x=w422, lower limit=w425) -> (In Range?=w427:bool)  [unwired: 1 out]
            n242 = case shown="False" w427 {
              tunnel: w424 -> [_ w431]
              tunnel: [w429 w430] -> w423
              tunnel: w422 -> [w428 _]
              frame False {
                n243 = local write "ultimo valor 2"(w428) -> ()
                n244 = Number To Decimal String(number=w428) -> (decimal integer string=w429:string)  [unwired: 1 in]
              }
              frame True {
                n245 = Number To Decimal String(number=w431) -> (decimal integer string=w430:string)  [unwired: 1 in]
              }
            }
          }
          frame True {
            n246 = Number To Decimal String(number=w432) -> (decimal integer string=w433:string)  [unwired: 1 in]
            "ultimo valor 2" <- w432
          }
        }
        n247 = Concatenate Strings(" FOCUS=" ("string"), w342, w338, " " ("string")) -> (w340:string)
        n248 = Number To Fractional String(number=w332, precision (6)=i16 1) -> (F-format string=w323:string)  [unwired: 2 in]
        n249 = Number To Fractional String(number=w331, precision (6)=i16 0) -> (F-format string=w322:string)  [unwired: 2 in]
        n250 = Number To Fractional String(number=w336, precision (6)=i16 1) -> (F-format string=w325:string)  [unwired: 2 in]
        n251 = String To Path(string=w305) -> (path=w303:path)
        n252 = call <vilib>:"Open_Create_Replace File.vi"("function (open:0)"=T1."open or create", "file path"=w303) -> ("error out"=w310:errorcluster, "refnum"=w313:refnum<file>)  [unwired: 6 in, 2 out]
        n253 = Concatenate Strings("WS_DEFAULT=" ("string"), w328, w321) -> (w320:string)
        n254 = Concatenate Strings("TEMP=" ("string"), w325, w321) -> (w319:string)
        n255 = Concatenate Strings("BAR=" ("string"), w323, w321) -> (w318:string)
        n256 = Concatenate Strings("HUM=" ("string"), w322, w321) -> (w317:string)
        n257 = Set File Position(refnum=w313, from (0:start)=enum16{"start", "end", "current"}."end" ("pos mode (0:2)"), error in=w310) -> (refnum out=w307:refnum<file>, error out=w306:errorcluster)  [unwired: 1 in]
        n258 = Concatenate Strings(w351, w330, w409, w330, w400, w330, w345, w330, w396, w330, w392, w330, w382, w330, w374, w330, w358, w330, w357, w340, w320, w319, w318, w317, "\r") -> (w302:string)
        n259 = disable-structure shown="Disabled" {
          disable-tunnel: w302 -> [w420 _]
          frame Disabled {
            n260 = global read "Global_Telescopio.vi" "AQUISICAO RESOURCE"() -> (w421:refnum<visa-resource-name>)
            n261 = call "TX.vi"("tx_buf"=w420, "VISA resource name"=w421) -> ()  [unwired: 1 in, 3 out]
          }
          frame Enabled {
          }
        }
        n262 = Write to Text File(file (use dialog)=w307, text=w302, error in=w306) -> (refnum out=w312:refnum<file>, error out=w311:errorcluster)  [unwired: 1 in, 1 out]
        n263 = Close File(refnum=w312, error in=w311) -> (error out=→"error out":errorcluster)  [unwired: 1 out]
      }
    }
    n264 = Wait Until Next ms Multiple(millisecond multiple=u32 100) -> ()  [unwired: 1 out]
    n265 = global read "Global_Telescopio.vi" "stop"() -> (w9:bool)
    "Maq Satus" <- w7
  }
